vi "Sound-Events2Case.vi"(2 "Sound Controls Old":T3, 3 "Sound Controls New":T3) -> (0 "Sound Cambio Array":T1(array[ring]), 1 "Sound Cambio?":bool)   [LabVIEW 2010]
uses:
  <vilib>/sound2/lvsound2.llb/Sound Data Format.ctl
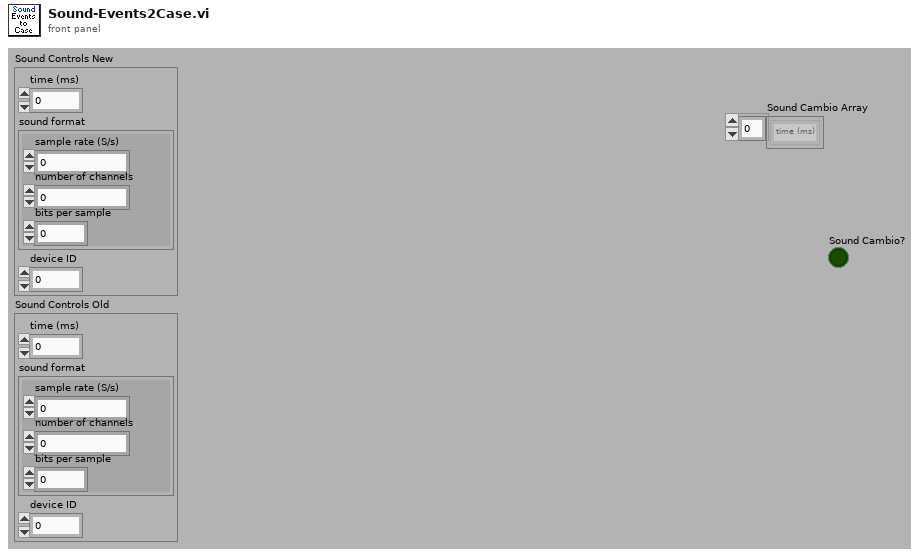
[diagram p1: front panel]
types:
  T1 = enum16{"time (ms)", "Sound Format", "Device ID", "Nothing"}[]
  T2 = typedef "Sound Data Format.ctl" = cluster{"sample rate (S/s)":dbl, "number of channels":i32, "bits per sample":i32}
  T3 = cluster{"time (ms)":dbl, "sound format":T2, "device ID":u32}
  T4 = enum16{"time (ms)", "Sound Format", "Device ID", "Nothing"}
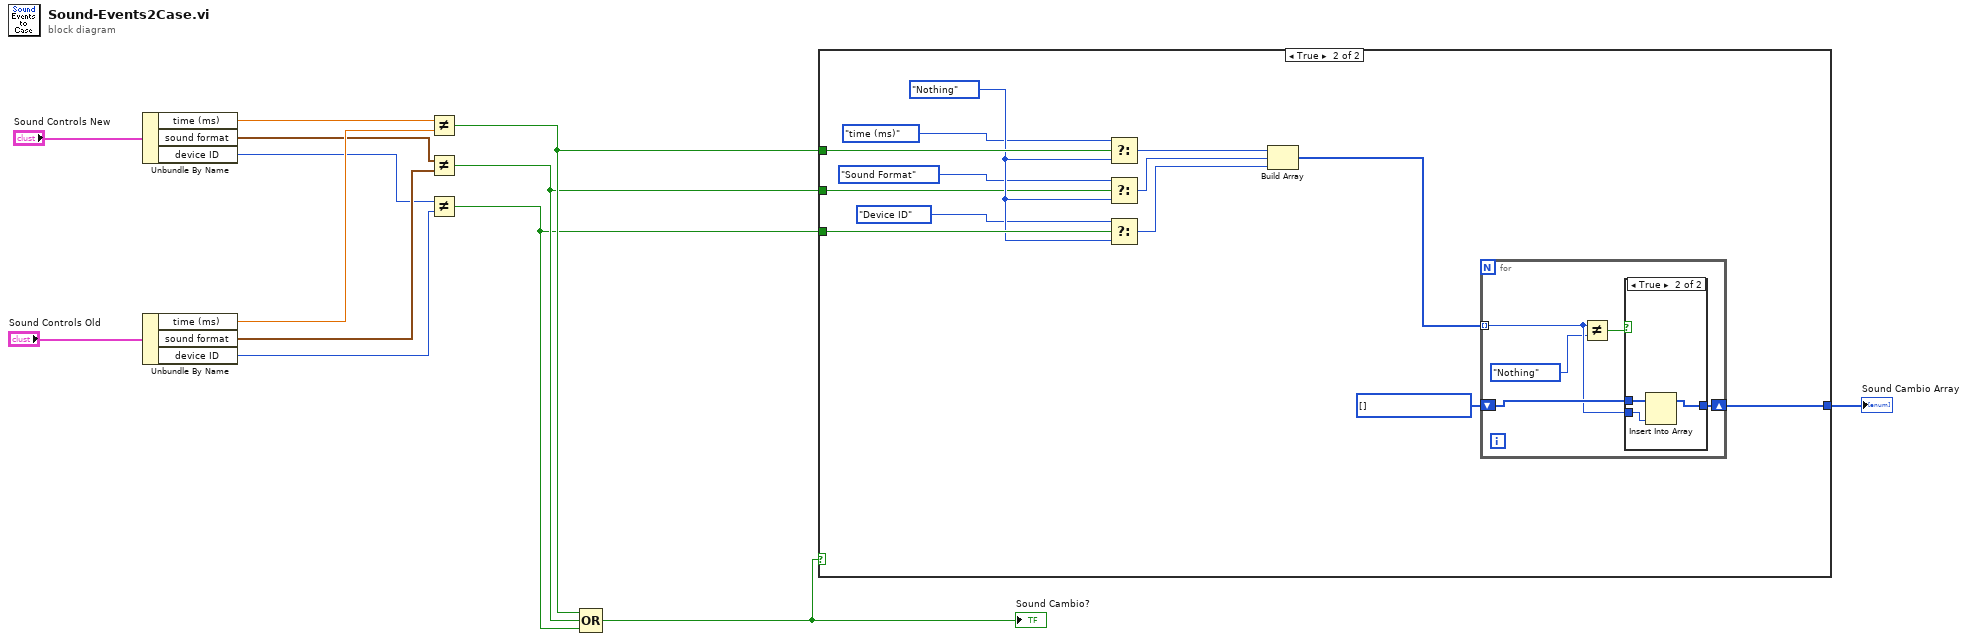
[diagram p0: block diagram]
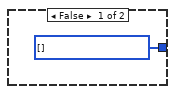
[diagram p2: hidden frame]
diagram:
  n1 = Unbundle By Name("Sound Controls New") -> ("time (ms)"=w13:dbl, "sound format"=w11:T2, "device ID"=w9:u32)
  n2 = Unbundle By Name("Sound Controls Old") -> ("time (ms)"=w12:dbl, "sound format"=w10:T2, "device ID"=w8:u32)
  n3 = Not Equal?(x=w13, y=w12) -> (x != y?=w7:bool)
  n4 = Not Equal?(x=w11, y=w10) -> (x != y?=w6:bool)
  n5 = Not Equal?(x=w9, y=w8) -> (x != y?=w5:bool)
  n6 = Compound Arithmetic op=OR(w7, w6, w5) -> (w2:bool)
  "Sound Cambio?" <- w2
  n7 = case shown="True" w2 {
    tunnel: w7 -> [_ w24]
    tunnel: w6 -> [_ w16]
    tunnel: w5 -> [_ w23]
    tunnel: [w14 w15] -> w1
    frame False {
      w14 = T1 [] items=["time (ms)", "Sound Format", "Device ID", "Nothing"]
    }
    frame True {
      w17 = T1 [] items=["time (ms)", "Sound Format", "Device ID", "Nothing"]
      w22 = T4."Nothing"
      n8 = Select(t=T4."time (ms)", s=w24, f=w22) -> (s? t:f=w27:T4)
      n9 = Select(t=T4."Sound Format", s=w16, f=w22) -> (s? t:f=w26:T4)
      n10 = Select(t=T4."Device ID", s=w23, f=w22) -> (s? t:f=w25:T4)
      n11 = Build Array(w27, w26, w25) -> (w21:T1)
      n12 = for {
        tunnel: w21 -> [w30] mode=indexing
        shift-right: [w29] -> w15
        shift-left: w17 -> [w31]
        n13 = Not Equal?(x=w30, y=T4."Nothing") -> (x != y?=w32:bool)
        n14 = case shown="True" w32 {
          tunnel: w31 -> [w33 w36]
          tunnel: w30 -> [_ w34]
          tunnel: [w33 w35] -> w29
          frame False {
          }
          frame True {
            n15 = Insert Into Array(array=w36, new element=w34) -> (w35:T1)  [unwired: 1 in]
          }
        }
      }
    }
  }
  "Sound Cambio Array" <- w1
